vi "Substitute Error.vi"(6 "Substitute?":bool=TRUE, 7 "LabVIEW Object":refnum<class>, 8 "error in (no error)":errorcluster, 9 "Error/Warning":bool=TRUE, 10 "Error Code":i32, 11 "Optional String":string) -> (0 "error out":errorcluster)   [LabVIEW 2026, in "TALOS.lvlib"]
doc: "This VI is useful for translate LabVIEW errors, that are meaningless if extrapolated from the context, to AEgIS-specific errors, easier to handle. This VI DOES NOTHING if no error are present in Error In: to generate an error in every circumstance please use Generate Error. BONUS: see at the end!\nIf in \"Error In\" an error is present, this VI substitute it (them, if multiples) with the error specified in Error Code. Setting Error/Warning to False generate a warning, and the Optional String get appeneded at the end of the error string. If an object is given in input, also its class name will be added in the error string. \nBONUS: if in LabVIEW Object a valid uService is wired, then the error(s) that gets substituted are logged in the Error Log."
uses:
  TALOS.lvlib
  Ancestor/Ancestor/Ancestor.lvclass/Ancestor.ctl
  FGV/Error Memory/Get Error Description.vi
  Get PC name.vi
  Ancestor/Ancestor/Read ID.vi
  Get Class Name.vi
  <vilib>/Utility/error.llb/Clear Errors.vi
  FGV/Error Memory/Error Memory Core.vi
  <vilib>/AdvancedString/Delimited String to 1D String Array.vi
  <vilib>/AdvancedString/Delimited String to 1D String Array (string).vi
  Circus Root Path.vi
  FGV/Error Memory/Error Crt Lvl checker.vi
  FGV/Error Memory/Error Memory Core.vi/40c8088d-b597-4017-91af-faa98e00292e.vi
  FGV/Error Memory/Error Memory Core.vi/d4a3ab98-063c-4e44-b43d-fbdcfe6c2be2.vi
  Global Memory.vi
  <vilib>/Utility/LVClass/Get LV Class Name.vi
  Is in Packed Library.vi
  TALOS Root path.vi
  Read CSV worksheet.vi
  Global Constants.vi
  <vilib>/Utility/error.llb/General Error Handler.vi
  Ancestor/Ancestor/Ancestor.lvclass
  <vilib>/Comparison/Equal/Equal Functor/Equal Functor.lvclass
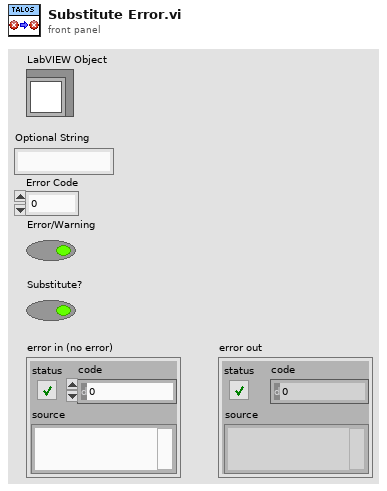
[diagram p1: front panel]
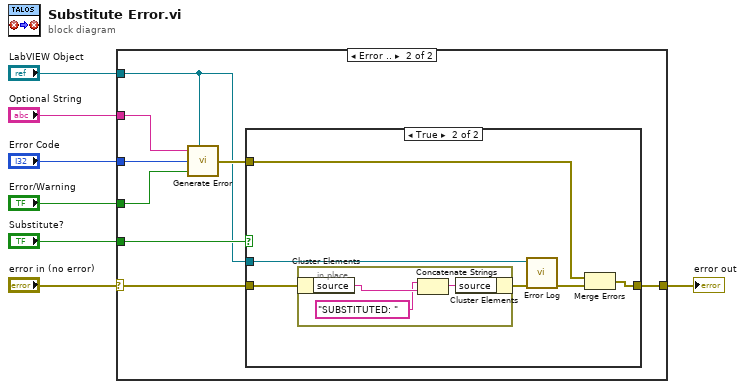
[diagram p0: block diagram]
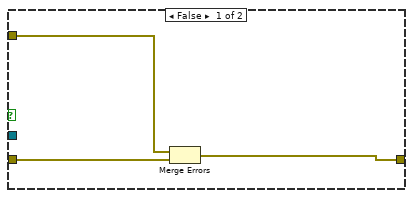
[diagram p3: hidden frame]
diagram:
  n1 = case shown="Error .." "error in (no error)" {
    selector: "error in (no error)" -> [w8 w12]
    tunnel: "Optional String" -> [_ w16]
    tunnel: "Error Code" -> [_ w15]
    tunnel: "Error/Warning" -> [_ w14]
    tunnel: [w8 w10] -> w3
    tunnel: "Substitute?" -> [_ w13]
    tunnel: "LabVIEW Object" -> [_ w9]
    frame No Error {
    }
    frame Error {
      n2 = call "Generate Error.vi"("Optional String"=w16, "Class"=w9, "Error Code"=w15, "Error/Warning"=w14) -> ("error out"=w11:errorcluster)  [unwired: 3 in]
      n3 = case shown="True" w13 {
        tunnel: w12 -> [w18 w24]
        tunnel: w11 -> [w19 w25]
        tunnel: [w17 w21] -> w10
        tunnel: w9 -> [_ w23]
        frame False {
          n4 = Merge Errors(w19, w18) -> (w17:errorcluster)
        }
        frame True {
          n5 = in-place {
            n6 = in-place-cluster #1(w24) -> ("source"=w27:string)
            n7 = Concatenate Strings("SUBSTITUTED: " ("string"), w27) -> (w28:string)
            n8 = in-place-cluster #1("source"=w28) -> (w22:errorcluster)
          }
          n9 = call "Error Log.vi"("error in (no error)"=w22, "Object in"=w23) -> ("error out"=w20:errorcluster)  [unwired: 9 in]
          n10 = Merge Errors(w25, w20) -> (w21:errorcluster)
        }
      }
    }
  }
  "error out" <- w3
